vi "fgv_AOwave.vi"(7 "cmd":T1, 8 "error in":errorcluster, 11 "signal in":waveform(dbl) caption="signal out") -> (0 "error out":errorcluster, 3 "signal out":waveform(dbl))   [LabVIEW 2019]
uses:
  _ctrl/rw.ctl
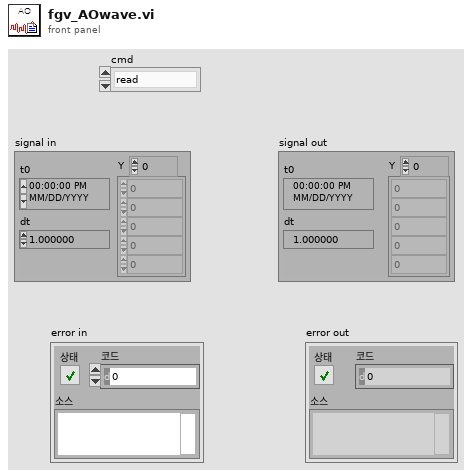
[diagram p1: front panel]
types:
  T1 = typedef "rw.ctl" = enum16{"read", "write"}
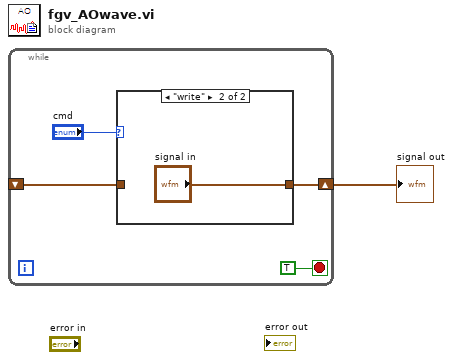
[diagram p0: block diagram]
diagram:
  n1 = while {
    shift-right: [w3] -> w1
    shift-left: _ -> [w2]
    stop <- TRUE stop-if-true
    n2 = case shown="\"write\"" "cmd" {
      tunnel: [w6 "signal in"] -> w3
      tunnel: w2 -> [w6 _]
      frame "read", Default {
      }
      frame "write" {
      }
    }
  }
  "signal out" <- w1
